vi "FeedbackDecode_20200902.vi"() -> ()   [LabVIEW 2016] (continued)
  T12 = cluster{"ExperimentDate":timestamp, "ImplantDate":timestamp, "CerebusFolder":string, "Experimenter":string, "PatientNumber":string, "DominantHand":string, "DeviceType":string, "DeviceSerial":string, "DeviceHemisphere":string, "DeviceRegion":string, "TaskType":string, "TaskComments":string, "RecordingComments":string, "GeneralObservations":string}
  T13 = typedef "FeedbackDecode_CogLoadClust.ctl" = cluster{"EEGTrigger":bool, "ConnectECG":bool, "TriggerECGwithTargets":bool, "SecondaryTask":bool, "MinTimeBetweenStimuli":dbl, "VariableTimeBetweenStimuli":dbl, "StimulusDuration":dbl}
  T14 = cluster{"[0]":u32, "[1]":u32, "[2]":u32, "[3]":u32}
  T15 = enum16{"---", "ReadMvnt", "WriteMvnt", "ReadEncode", "WriteEncode", "ReadDecode", "WriteDecode"}
  T16 = enum16{"Initialize", "Acquire Start", "Acquire Response", "Finalize"}
  T17 = enum8{"Enabled", "Disabled", "Disabled and Grayed Out"}
  T18 = enum16{"---", "Bakeoff11", "Bakeoff21", "Bakeoff31", "Bakeoff32", "LukeEmpty", "MPLEmpty", "MPLUnknown", "MPLBasic", "MPLTarg", "LukeBasic"}
  T19 = enum16{"Initialize", "Wait", "BuildInitStr", "BuildKalmanStr", "BuildStimStr", "BuildEMGStr", "GetEvent", "SendEvent", "ContIO", "LoadTrainFile", "CopyTraining", "Close"}
  T20 = cluster{"LV":cluster{"Name":string, "IP":string}, "ML":cluster{"Name":string, "IP":string}}
  T21 = enum32{"Invalid", "Standard", "Closed", "Hidden", "Minimized", "Maximized"}
  T22 = enum16{"open", "replace", "create", "open or create", "replace or create", "replace or create with confirmation"}
  T23 = enum16{"MSMS", "Bakeoff11", "Bakeoff21", "Bakeoff31", "Bakeoff32", "Bakeoff32_Ball", "Bakeoff32_Checkers", "Bakeoff32_Pen", "FragileBlock"}
  T24 = cluster{"MvntMat":dbl[][], "MvntName":string, "Tracking":enum8{"False", "True", "Mixed"}, "Radius":dbl}[]
  T25 = cluster{"Boolean 1":bool, "Boolean 2":bool, "Boolean 3":bool, "Boolean 4":bool, "Boolean 5":bool, "Boolean 6":bool, "Boolean 7":bool, "Boolean 8":bool, "Boolean 9":bool, "Boolean 10":bool, "Boolean 11":bool, "Boolean 12":bool, "Boolean 13":bool, "Boolean 14":bool, "Boolean 15":bool, "Boolean 16":bool, "Boolean 17":bool, "Boolean 18":bool, "Boolean 19":bool, "Boolean 20":bool, "Boolean 21":bool, "Boolean 22":bool, "Boolean 23":bool, "Boolean 24":bool, "Boolean 25":bool, "Boolean 26":bool, "Boolean 27":bool, "Boolean 28":bool, "Boolean 29":bool, "Boolean 30":bool, "Boolean 31":bool, "Boolean 32":bool, "Boolean 33":bool, "Boolean 34":bool, "Boolean 35":bool, "Boolean 36":bool, "Boolean 37":bool, "Boolean 38":bool, "Boolean 39":bool, "Boolean 40":bool, "Boolean 41":bool, "Boolean 42":bool, "Boolean 43":bool, "Boolean 44":bool, "Boolean 45":bool, "Boolean 46":bool, "Boolean 47":bool, "Boolean 48":bool, "Boolean 49":bool, "Boolean 50":bool, "Boolean 51":bool, "Boolean 52":bool, "Boolean 53":bool, "Boolean 54":bool, "Boolean 55":bool, "Boolean 56":bool, "Boolean 57":bool, "Boolean 58":bool, "Boolean 59":bool, "Boolean 60":bool, "Boolean 61":bool, "Boolean 62":bool, "Boolean 63":bool, "Boolean 64":bool, "Boolean 65":bool, "Boolean 66":bool, "Boolean 67":bool, "Boolean 68":bool, "Boolean 69":bool, "Boolean 70":bool, "Boolean 71":bool, "Boolean 72":bool, "Boolean 73":bool, "Boolean 74":bool, "Boolean 75":bool, "Boolean 76":bool, "Boolean 77":bool, "Boolean 78":bool, "Boolean 79":bool, "Boolean 80":bool, "Boolean 81":bool, "Boolean 82":bool, "Boolean 83":bool, "Boolean 84":bool, "Boolean 85":bool, "Boolean 86":bool, "Boolean 87":bool, "Boolean 88":bool, "Boolean 89":bool, "Boolean 90":bool, "Boolean 91":bool, "Boolean 92":bool, "Boolean 93":bool, "Boolean 94":bool, "Boolean 95":bool, "Boolean 96":bool, "Boolean 97":bool, "Boolean 98":bool, "Boolean 99":bool, "Boolean 100":bool}[]
  T26 = cluster{"[0]":dbl, "[1]":dbl, "[2]":dbl, "[3]":dbl, "[4]":dbl, "[5]":dbl, "[6]":dbl, "[7]":dbl, "[8]":dbl, "[9]":dbl, "[10]":dbl, "[11]":dbl}
  T27 = typedef "XDNodeRunTimeDep.lvlib/timing_clust.ctl" = cluster{"Expected End [f-1]":u64, "Actual End [f-1]":u64, "Finished Late? [f-1]":bool, "Expected End [i-1]":u64, "Actual End [i-1]":u64, "Finished Late? [i-1]":bool, "Expected Start [i]":u64, "Actual Start [i]":u64, "Expected Start [f]":u64, "Actual Start [f]":u64, "Source Name":string, "Structure Name":string, "Period":i64, "Deadline":i64, "Offset":i64, "Start":i64, "Priority":i32, "Timeout":i32, "Mode":T28, "Wakeup Reason":T29, "Error":errorcluster, "Source Type":string, "Secondary Source Type":string, "Global End Time":u64, "Global Start Time":u64, "Frame Duration":u64, "Iteration Duration":u64, "Assigned CPU":i32, "I/O Scan Engine Mode":u32}
  T28 = typedef "XDNodeRunTimeDep.lvlib/nitl_modes.ctl" = enum32{"No Change", "Process missed periods, maintain original phase", "Discard missed periods, maintain original phase", "Process missed periods, ignore original phase", "Discard missed periods, ignore original phase"}
  T29 = typedef "XDNodeRunTimeDep.lvlib/wakeup.ctl" = enum32{"Normal", "Aborted", "Asynchronous wakeup", "Timing source error", "Timed loop error", "Timeout"}
  T30 = enum16{"MSMS", "BakeOff1", "BakeOff2", "BakeOff3"}
  T31 = typedef "LVPositionTypeDef.ctl" = cluster{"Left":i32, "Top":i32}
  T32 = typedef "LVBoundsTypeDef.ctl" = cluster{"Width":u32, "Height":u32}
  T33 = cluster{cluster{"[0]":u32, "[1]":u32, "[2]":u32, "[3]":u32}, "HMSize":cluster{"NumCol":dbl, "NumRows":dbl}}
  T34 = cluster{"Left":i32, "Top":i32, "Width":u32, "Height":u32}
  T35 = cluster{"Name":string, "Type":string, "ID":string, "Num":string, "COM":dbl[], "Offset":dbl[], "RotationAxis":dbl[], "OrientationMatrix":dbl[][], "MinAngle":dbl, "MaxAngle":dbl, "InboardID":string, "InboardNum":string, "InboardCOM":dbl[], "OutboardID":string, "OutboardNum":string, "OutboardCOM":dbl[]}[]
  T36 = cluster{"ModelName":string, "Value":dbl[][], "CompNames":string[]}
  T37 = enum16{"Off", "Training", "Decode", "COB", "LEAP"}
  T38 = cluster{"ContMvntVal[0]":dbl, "ContMvntVal[1]":dbl, "ContMvntVal[2]":dbl, "ContMvntVal[3]":dbl, "ContMvntVal[4]":dbl, "ContMvntVal[5]":dbl, "ContMvntVal[6]":dbl, "ContMvntVal[7]":dbl, "ContMvntVal[8]":dbl, "ContMvntVal[9]":dbl, "ContMvntVal[10]":dbl, "ContMvntVal[11]":dbl}
  T39 = cluster{"ContTargetVal[0]":dbl, "ContTargetVal[1]":dbl, "ContTargetVal[2]":dbl, "ContTargetVal[3]":dbl, "ContTargetVal[4]":dbl, "ContTargetVal[5]":dbl, "ContTargetVal[6]":dbl, "ContTargetVal[7]":dbl, "ContTargetVal[8]":dbl, "ContTargetVal[9]":dbl, "ContTargetVal[10]":dbl, "ContTargetVal[11]":dbl}
  T40 = cluster{"LoopTimings":cluster{"MLCalcTime":dbl, "MLTotalTime":dbl}, "Kalman":cluster{"Thumb":dbl, "Index":dbl, "Middle":dbl, "Ring":dbl, "Little":dbl, "ThumbInt":dbl, "IndexInt":dbl, "RingInt":dbl, "LittleInt":dbl, "Wrist":dbl, "WristYaw":dbl, "WristRoll":dbl}, "Kinematics":cluster{"Thumb":dbl, "Index":dbl, "Middle":dbl, "Ring":dbl, "Little":dbl, "ThumbInt":dbl, "IndexInt":dbl, "RingInt":dbl, "LittleInt":dbl, "Wrist":dbl, "WristYaw":dbl, "WristRoll":dbl}, "ElectRates":dbl[], "SelWfs":dbl[][], "TrainCnt":dbl, "EMGPwr":dbl[], "SelData":cluster{dbl, dbl, "RasterOut":dbl[]}[], "SelRate":cluster{"CurIdx":dbl, dbl, "RasterOut":dbl[]}[], "SelKin":cluster{dbl, dbl, "RasterOut":dbl[]}[], "NIPTime":dbl, "VREID":i16, "StimWf":dbl[], "RawDecodeOutput":dbl[], "TASKA IR sensors":dbl[], "TASKA baro sensors":dbl[]}
  T41 = cluster{"Thumb":dbl, "Index":dbl, "Middle":dbl, "Ring":dbl, "Little":dbl, "ThumbInt":dbl, "IndexInt":dbl, "RingInt":dbl, "LittleInt":dbl, "Wrist":dbl, "WristYaw":dbl, "WristRoll":dbl}
  T42 = cluster{"Delay":dbl, "Rise":dbl, "Hold":dbl, "Trial":dbl}
  T43 = enum16{"Position", "Latching", "Leaky", "Velocity"}[]
  T44 = enum16{"Standard", "Mean", "Refit", "LinSVReg", "NonLinSVReg", "PCA", "DWPRR", "AdaptKF", "NN", "NN_python", "AdaptKF2", "KF_Short_Goal"}
  T45 = typedef "LVPoint32TypeDef.ctl" = cluster{"Horizontal":i32, "Vertical":i32}
  T46 = cluster{"KGain":sgl[][], "KMvnts":cluster{"Thumb":bool, "Index":bool, "Middle":bool, "Ring":bool, "Little":bool, "ThumbInt":bool, "IndexInt":bool, "RingInt":bool, "LittleInt":bool, "WristPitch":bool, "WristYaw":bool, "WristRoll":bool}, "KThresh":sgl[][], "CtrlMode":enum16{"Position", "Latching", "Leaky", "Velocity"}[], "CtrlSpd":sgl[]}
  T47 = enum16{"RMS Single", "RMS All", "RMS Auto", "Volt Single", "Volt All"}
  T48 = cluster{"[0]":bool, "[1]":bool, "[2]":bool, "[3]":bool, "[4]":bool, "[5]":bool, "[6]":bool, "[7]":bool, "[8]":bool, "[9]":bool, "[10]":bool, "[11]":bool, "[12]":bool, "[13]":bool, "[14]":bool, "[15]":bool, "[16]":bool, "[17]":bool, "[18]":bool, "[19]":bool, "[20]":bool, "[21]":bool, "[22]":bool, "[23]":bool, "[24]":bool, "[25]":bool, "[26]":bool, "[27]":bool, "[28]":bool, "[29]":bool, "[30]":bool, "[31]":bool, "[32]":bool, "[33]":bool, "[34]":bool, "[35]":bool, "[36]":bool, "[37]":bool, "[38]":bool, "[39]":bool, "[40]":bool, "[41]":bool, "[42]":bool, "[43]":bool, "[44]":bool, "[45]":bool, "[46]":bool, "[47]":bool, "[48]":bool, "[49]":bool, "[50]":bool, "[51]":bool, "[52]":bool, "[53]":bool, "[54]":bool, "[55]":bool, "[56]":bool, "[57]":bool, "[58]":bool, "[59]":bool, "[60]":bool, "[61]":bool, "[62]":bool, "[63]":bool, "[64]":bool, "[65]":bool, "[66]":bool, "[67]":bool, "[68]":bool, "[69]":bool, "[70]":bool, "[71]":bool, "[72]":bool, "[73]":bool, "[74]":bool, "[75]":bool, "[76]":bool, "[77]":bool, "[78]":bool, "[79]":bool, "[80]":bool, "[81]":bool, "[82]":bool, "[83]":bool, "[84]":bool, "[85]":bool, "[86]":bool, "[87]":bool, "[88]":bool, "[89]":bool, "[90]":bool, "[91]":bool, "[92]":bool, "[93]":bool, "[94]":bool, "[95]":bool, "[96]":bool, "[97]":bool, "[98]":bool, "[99]":bool}
  T49 = cluster{"[0]":bool, "[1]":bool, "[2]":bool, "[3]":bool, "[4]":bool, "[5]":bool, "[6]":bool, "[7]":bool, "[8]":bool, "[9]":bool, "[10]":bool, "[11]":bool, "[12]":bool, "[13]":bool, "[14]":bool, "[15]":bool, "[16]":bool, "[17]":bool, "[18]":bool, "[19]":bool, "[20]":bool, "[21]":bool, "[22]":bool, "[23]":bool, "[24]":bool, "[25]":bool, "[26]":bool, "[27]":bool, "[28]":bool, "[29]":bool, "[30]":bool, "[31]":bool, "[32]":bool, "[33]":bool, "[34]":bool, "[35]":bool, "[36]":bool, "[37]":bool, "[38]":bool, "[39]":bool, "[40]":bool, "[41]":bool, "[42]":bool, "[43]":bool, "[44]":bool, "[45]":bool, "[46]":bool, "[47]":bool, "[48]":bool, "[49]":bool, "[50]":bool, "[51]":bool, "[52]":bool, "[53]":bool, "[54]":bool, "[55]":bool, "[56]":bool, "[57]":bool, "[58]":bool, "[59]":bool, "[60]":bool, "[61]":bool, "[62]":bool, "[63]":bool, "[64]":bool, "[65]":bool, "[66]":bool, "[67]":bool, "[68]":bool, "[69]":bool, "[70]":bool, "[71]":bool, "[72]":bool, "[73]":bool, "[74]":bool, "[75]":bool, "[76]":bool, "[77]":bool, "[78]":bool, "[79]":bool}
  T50 = enum16{"Position", "Latching", "Leaky", "Velocity"}
  T51 = cluster{"Shift":bool, "Ctrl":bool, "Alt":bool, "Cmd":bool, "Opt":bool}
  T52 = cluster{"Region":bool, "Receptor":bool, "Electrode":bool, "Min Amp":bool, "Max Amp":bool, "Min Freq":bool, "Max Freq":bool, "Duration":bool}
  T53 = typedef "eventvkey.ctl" = enum16{"ASCII", "Enter", "Return", "Shift", "Ctrl", "Alt", "Cmd", "Opt", "Caps", "NumLock", "Clear", "Break", "Up", "Down", "Left", "Right", "Insert", "Delete", "Home", "End", "PageUp", "PageDown", "Escape", "Help", "Pause", "ScrollLock", "F1", "F2", "F3", "F4", "F5", "F6", "F7", "F8", "F9", "F10", "F11", "F12", "F13", "F14", "F15", "F16", "F17", "F18", "F19", "F20", "F21", "F22", "F23", "F24", "Play", "VolumeUp", "VolumeDown", "Mute", "Two Byte Char"}
  T54 = cluster{"Boolean 1":bool, "Boolean 2":bool, "Boolean 3":bool, "Boolean 4":bool, "Boolean 5":bool, "Boolean 6":bool, "Boolean 7":bool, "Boolean 8":bool, "Boolean 9":bool, "Boolean 10":bool, "Boolean 11":bool, "Boolean 12":bool, "Boolean 13":bool, "Boolean 14":bool, "Boolean 15":bool, "Boolean 16":bool, "Boolean 17":bool, "Boolean 18":bool, "Boolean 19":bool, "Boolean 20":bool, "Boolean 21":bool, "Boolean 22":bool, "Boolean 23":bool, "Boolean 24":bool, "Boolean 25":bool, "Boolean 26":bool, "Boolean 27":bool, "Boolean 28":bool, "Boolean 29":bool, "Boolean 30":bool, "Boolean 31":bool, "Boolean 32":bool, "Boolean 33":bool, "Boolean 34":bool, "Boolean 35":bool, "Boolean 36":bool, "Boolean 37":bool, "Boolean 38":bool, "Boolean 39":bool, "Boolean 40":bool, "Boolean 41":bool, "Boolean 42":bool, "Boolean 43":bool, "Boolean 44":bool, "Boolean 45":bool, "Boolean 46":bool, "Boolean 47":bool, "Boolean 48":bool, "Boolean 49":bool, "Boolean 50":bool, "Boolean 51":bool, "Boolean 52":bool, "Boolean 53":bool, "Boolean 54":bool, "Boolean 55":bool, "Boolean 56":bool, "Boolean 57":bool, "Boolean 58":bool, "Boolean 59":bool, "Boolean 60":bool, "Boolean 61":bool, "Boolean 62":bool, "Boolean 63":bool, "Boolean 64":bool, "Boolean 65":bool, "Boolean 66":bool, "Boolean 67":bool, "Boolean 68":bool, "Boolean 69":bool, "Boolean 70":bool, "Boolean 71":bool, "Boolean 72":bool, "Boolean 73":bool, "Boolean 74":bool, "Boolean 75":bool, "Boolean 76":bool, "Boolean 77":bool, "Boolean 78":bool, "Boolean 79":bool, "Boolean 80":bool, "Boolean 81":bool, "Boolean 82":bool, "Boolean 83":bool, "Boolean 84":bool, "Boolean 85":bool, "Boolean 86":bool, "Boolean 87":bool, "Boolean 88":bool, "Boolean 89":bool, "Boolean 90":bool, "Boolean 91":bool, "Boolean 92":bool, "Boolean 93":bool, "Boolean 94":bool, "Boolean 95":bool, "Boolean 96":bool, "Boolean 97":bool, "Boolean 98":bool, "Boolean 99":bool, "Boolean 100":bool}
  T55 = cluster{"[0]":bool, "[1]":bool, "[2]":bool, "[3]":bool, "[4]":bool, "[5]":bool, "[6]":bool, "[7]":bool, "[8]":bool, "[9]":bool, "[10]":bool, "[11]":bool, "[12]":bool, "[13]":bool, "[14]":bool, "[15]":bool, "[16]":bool, "[17]":bool, "[18]":bool, "[19]":bool, "[20]":bool, "[21]":bool, "[22]":bool, "[23]":bool, "[24]":bool, "[25]":bool, "[26]":bool, "[27]":bool, "[28]":bool, "[29]":bool, "[30]":bool, "[31]":bool, "[32]":bool, "[33]":bool, "[34]":bool, "[35]":bool, "[36]":bool, "[37]":bool, "[38]":bool, "[39]":bool, "[40]":bool, "[41]":bool, "[42]":bool, "[43]":bool, "[44]":bool, "[45]":bool, "[46]":bool, "[47]":bool, "[48]":bool, "[49]":bool, "[50]":bool, "[51]":bool, "[52]":bool, "[53]":bool, "[54]":bool, "[55]":bool, "[56]":bool, "[57]":bool, "[58]":bool, "[59]":bool, "[60]":bool, "[61]":bool, "[62]":bool, "[63]":bool, "[64]":bool, "[65]":bool, "[66]":bool, "[67]":bool, "[68]":bool, "[69]":bool, "[70]":bool, "[71]":bool, "[72]":bool, "[73]":bool, "[74]":bool, "[75]":bool, "[76]":bool, "[77]":bool, "[78]":bool, "[79]":bool, "[80]":bool, "[81]":bool, "[82]":bool, "[83]":bool, "[84]":bool, "[85]":bool, "[86]":bool, "[87]":bool, "[88]":bool, "[89]":bool, "[90]":bool, "[91]":bool, "[92]":bool, "[93]":bool, "[94]":bool, "[95]":bool, "[96]":bool, "[97]":bool, "[98]":bool, "[99]":bool}[]
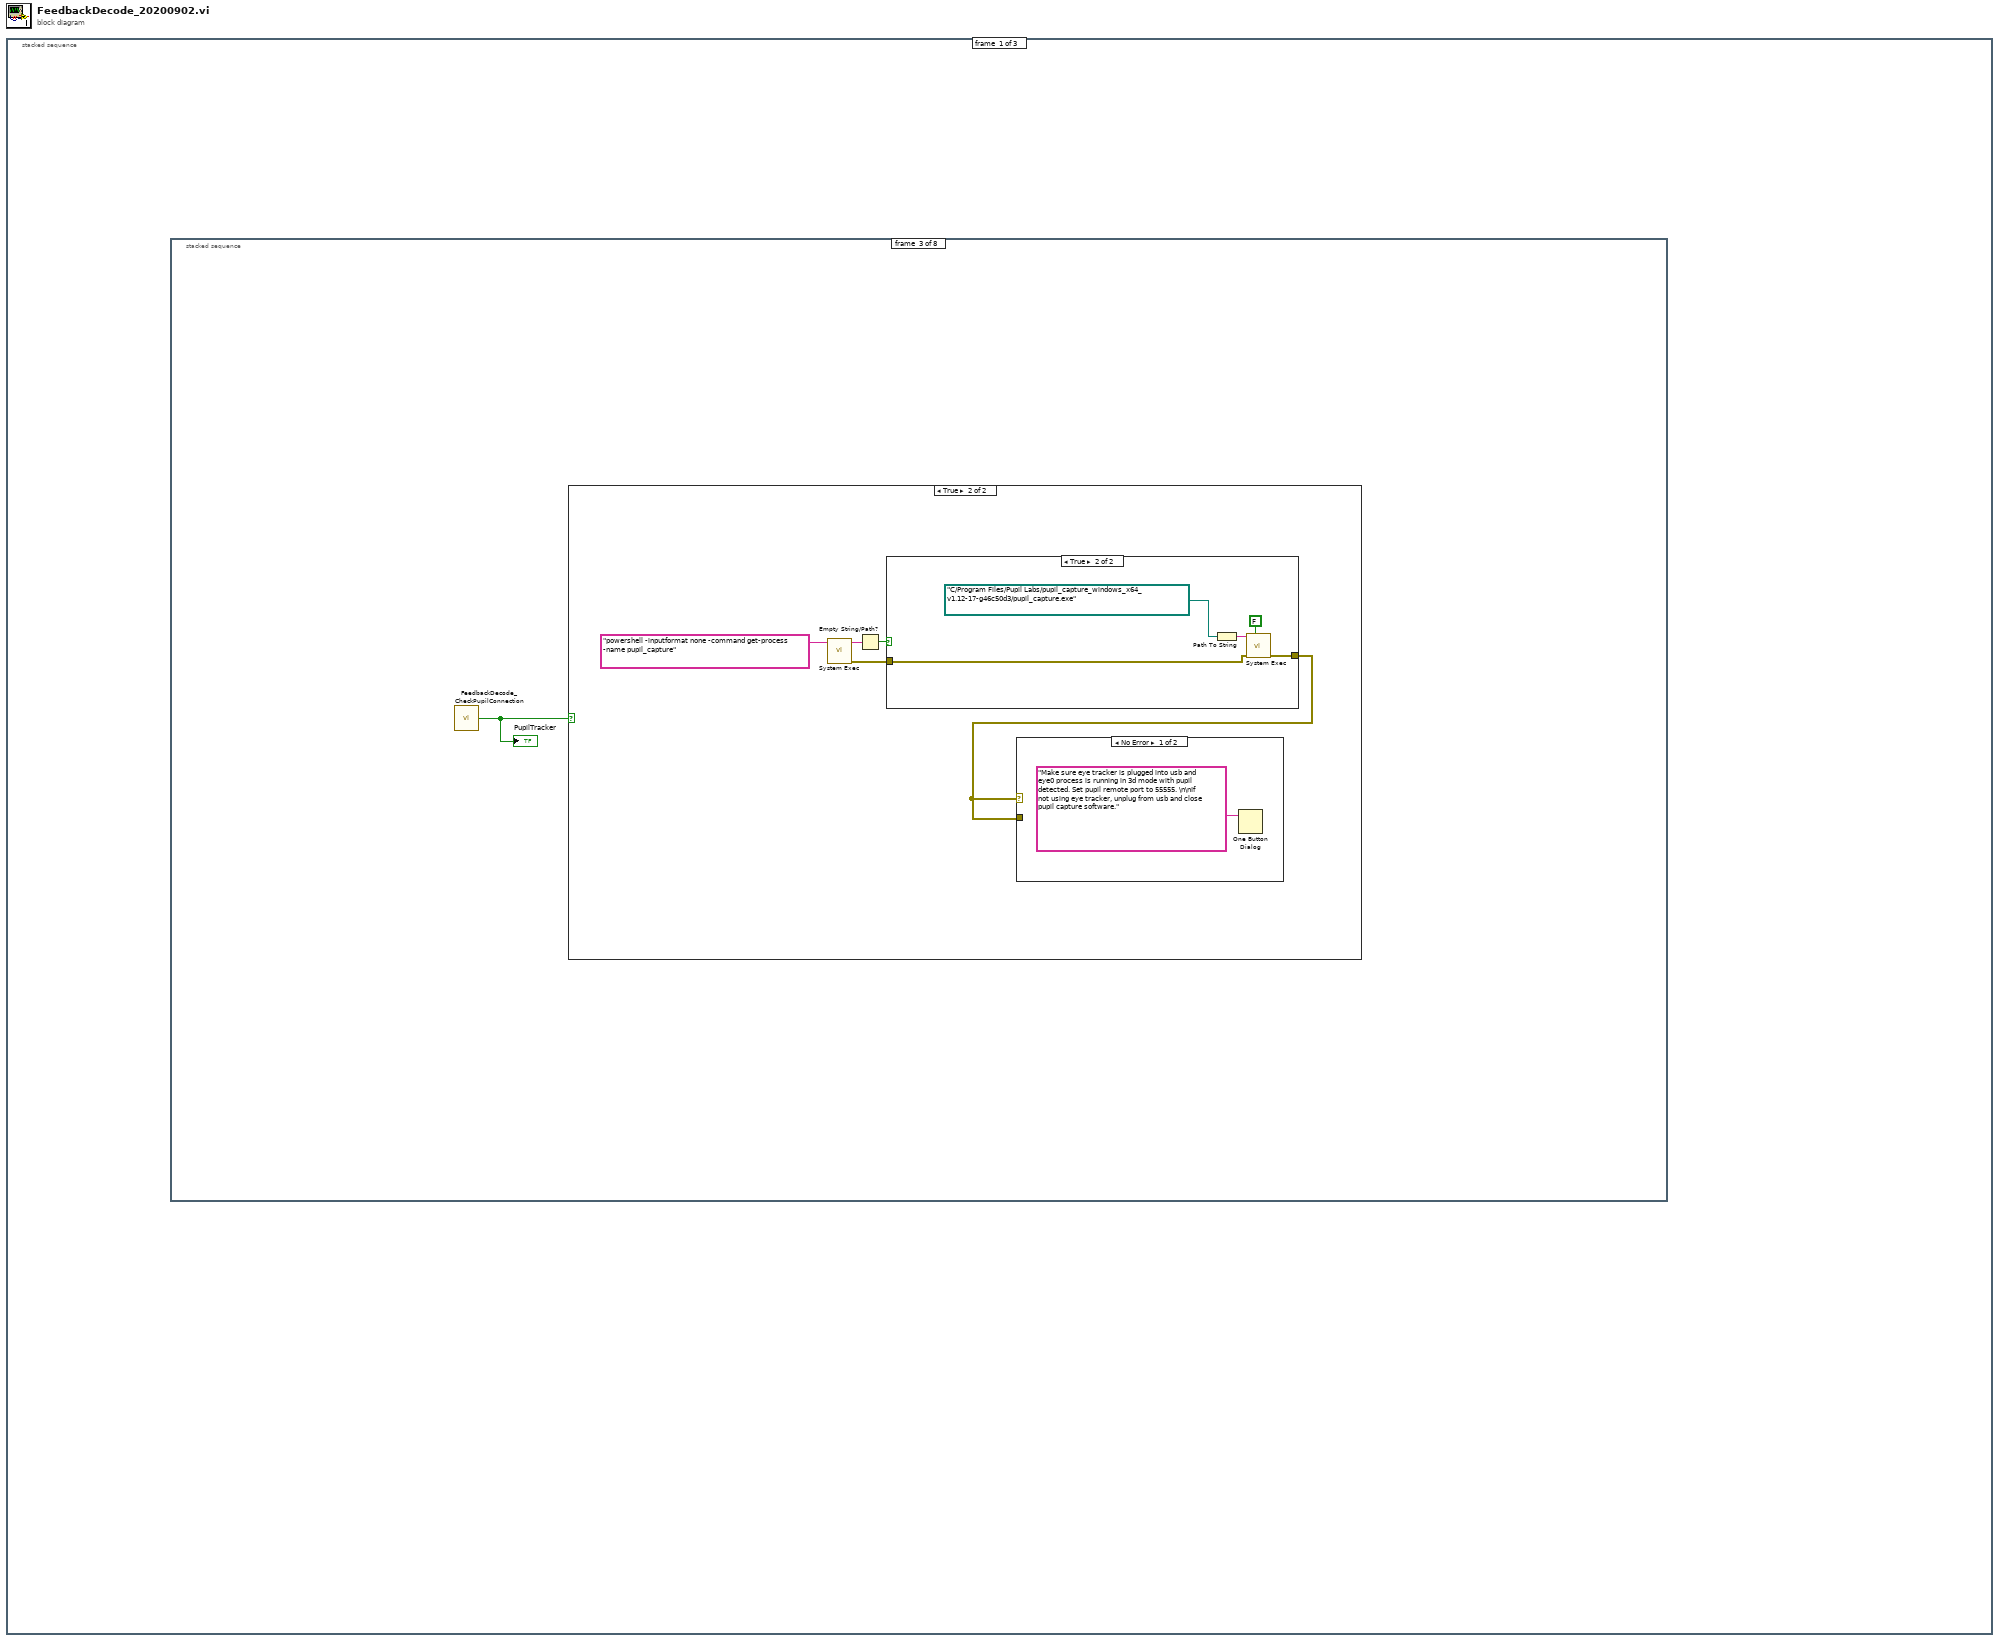
[diagram p0: block diagram]
diagram:
  n1 = stacked-sequence {
    frame #0 {
      n2 = stacked-sequence {
        frame #0 {
          w43 = FALSE ("Finished")
          w50 = 0.0  # MvntEvnt
          w66 = u64 0 ("BaseCnt1")
          w153 = enum16{"Initialize", "Reset", "Run"}."Initialize" ("Mode")
          w139 = "" ("TrialTypeStr")
          w120 = path "C:/Users/Administrator/Code/General/Databases/PatientDatabase.udl" ("DatabaseUDL")
          # "Is shared enabled?"
          # "TASKA"
          # "for analog sensors"
          n3 = local write "TASKASharedControlBeta"(0.0 ("TASKASharedControlBeta")) -> ()
          n4 = local write "Beta Mode"("Fixed" ("Beta Mode")) -> ()
          n5 = local write "Computer Goal"("Close" ("Computer Goal")) -> ()
          n6 = local write "TASKA Shared Control"(FALSE ("TASKA Shared Control")) -> ()
          n7 = property on="MedianHM" class="Pict"() -> ("Position"=w117:T31, "Draw Area Size"=w116:T32)  [unwired: 2 in, 2 out]
          n8 = property on="UlnarHM" class="Pict"() -> ("Position"=w112:T31, "Draw Area Size"=w113:T32)  [unwired: 2 in, 2 out]
          n9 = property on="EMGHM" class="Pict"() -> ("Position"=w98:T31, "Draw Area Size"=w97:T32)  [unwired: 2 in, 2 out]
          n10 = Initialize Array(0.0 ("element"), 496 ("dimension size")) -> (w52:dbl[])
          n11 = Cluster To Array(cluster=w117) -> (array=w146:i32[])
          n12 = Cluster To Array(cluster=w116) -> (array=w147:u32[])
          n13 = Cluster To Array(cluster=w112) -> (array=w111:i32[])
          n14 = Cluster To Array(cluster=w113) -> (array=w110:u32[])
          n15 = Cluster To Array(cluster=w98) -> (array=w99:i32[])
          n16 = Cluster To Array(cluster=w97) -> (array=w100:u32[])
          n17 = call "FeedbackDecode_AllEMGHM.vi"("Intensities"=w52, "Mode"=enum16{"Initialize", "Run"}."Initialize") -> ()  [unwired: 2 in]
          n18 = property on="Finished" class="Bool (strict)"("DisabledEnum"=T17."Disabled and Grayed Out" ("Disabled"), "Value"=w43, "Blinking"=w43) -> ()  [unwired: 2 in, 2 out]
          n19 = Build Array (concatenate)(w146, w147) -> (w148:u32[])
          n20 = Build Array (concatenate)(w111, w110) -> (w109:u32[])
          n21 = Build Array (concatenate)(w99, w100) -> (w101:u32[])
          n22 = mathscript code="GridArray = reshape(rot90(reshape(1:100,10,10),-1),1,100);"() -> ("GridArray"=→"UEAHMIdx":i32[])  [unwired: 1 in, 1 out]
          n23 = property on="ParamsTable" class="Arr (strict)"() -> ("Index Values"=w79:u32[], "Left"=w71:i32, "Width"=w70:u32)  [unwired: 2 in, 2 out]
          n24 = Array To Cluster(array=w148) -> (cluster=w149:T14)
          "MedianPos" <- w149
          n25 = Array To Cluster(array=w109) -> (cluster=w105:T14)
          "UlnarPos" <- w105
          n26 = Array To Cluster(array=w101) -> (cluster=w96:T14)
          "EMGPos" <- w96
          n27 = for {
            N: 2 -> [_]
            tunnel: [w178] -> w41 mode=indexing
            i -> [w177]
            n28 = case shown="0, Default" w177 {
              tunnel: [w179 w183] -> w178
              frame 0, Default {
                n29 = vi-ref "FeedbackDecode_PickROI.vi"() -> (w182:refnum<vi>)
                n30 = invoke class="VI" method="FP.Open"(reference=w182, "Activate"=TRUE ("Activate?"), "State"=T21."Hidden") -> (reference out=w179:refnum<vi>)  [unwired: 2 in, 4 out]
              }
              frame 1 {
                n31 = vi-ref "FeedbackDecode_PickROI_Adv.vi"() -> (w186:refnum<vi>)
                n32 = invoke class="VI" method="FP.Open"(reference=w186, "Activate"=TRUE ("Activate?"), "State"=T21."Hidden") -> (reference out=w183:refnum<vi>)  [unwired: 2 in, 4 out]
              }
            }
          }
          "RespRefArray" <- w41
          n33 = stacked-sequence {
            frame #0 {
              w169 = FALSE ("TASKA Reset Success")
              n34 = local write "TASKA Reset Success"(w169) -> ()
              n35 = local write "TASKA Reset Break"(w169) -> ()
              n36 = local write "TASKA Timer"(w169) -> ()
            }
            frame #1 {
              n37 = property on="TASKA Timer" class="Bool (strict)"("DisabledEnum"=T17."Enabled" ("Disabled")) -> ()  [unwired: 2 in, 2 out]
            }
          }
          n38 = Bundle(w149, "HMSize"="HMSize") -> (w150:T33)  [unwired: 1 in]
          n39 = Bundle(w105, "HMSize"="HMSize") -> (w106:T33)  [unwired: 1 in]
          n40 = Bundle(w96, "HMSize"="HMSize") -> (w104:T33)  [unwired: 1 in]
          n41 = call "FeedbackDecode_PlotHeatmap.vi"("InitCluster"=w150, "Instance"=0, "Mode"=enum16{"Initialize", "Run", "Mouse"}."Initialize") -> ("Pic"=→"MedianHM":picture, "CurrPos"=w90:i32)  [unwired: 3 in]
          "SelElect" <- w90
          n42 = call "FeedbackDecode_PlotHeatmap.vi"("InitCluster"=w106, "Instance"=1, "Mode"=enum16{"Initialize", "Run", "Mouse"}."Initialize") -> ("Pic"=→"UlnarHM":picture)  [unwired: 3 in, 1 out]
          n43 = call "FeedbackDecode_PlotHeatmap.vi"("InitCluster"=w104, "Instance"=2, "Mode"=enum16{"Initialize", "Run", "Mouse"}."Initialize") -> ("Pic"=→"EMGHM":picture)  [unwired: 3 in, 1 out]
          n44 = property on="Sel" class="Arr (strict)"("Index Values"=w79) -> ()  [unwired: 2 in, 2 out]
          n45 = Bundle("Left"=w71, "Width"=w70) -> (→"ParamsTableLoc":cluster{"Left":i32, "Width":u32})  [unwired: 1 in]
          n46 = disable-structure shown="Disabled" {
            frame Disabled {
              n47 = vi-ref "FeedbackDecode_MSMS2DEKA.vi"() -> (w176:refnum<vi>)
              n48 = invoke class="VI" method="FP.Open"(reference=w176, "Activate"=FALSE ("Activate?"), "State"=T21."Minimized") -> ()  [unwired: 2 in, 5 out]
            }
            frame Enabled {
            }
          }
          n49 = property on="KUEA" class="Clust (strict)"() -> ("Left"=w164:i32, "Top"=w163:i32, "Width"=w162:u32, "Height"=w161:u32)  [unwired: 2 in, 2 out]
          n50 = for {
            N: 80 -> [_]
            tunnel: [w190] -> w94 mode=indexing
            i -> [w191]
            n51 = Increment(x=w191) -> (x+1=w190:i32)
          }
          "EMGHMIdx" <- w94
          n52 = Initialize Array(0.0 ("element"), 100 ("dimension size")) -> (→"StimArray":dbl[])
          n53 = property class="VI"() -> ("Name"=→"TaskType":string)  [unwired: 2 in, 2 out]
          n54 = Bundle("Left"=w164, "Top"=w163, "Width"=w162, "Height"=w161) -> (w160:T34)  [unwired: 1 in]
          "HoverPicPos" <- w160
          n55 = call <vilib>:"Application Directory.vi"() -> ("Application Directory"=w29:path)
          n56 = call <vilib>:"Check if File or Folder Exists.vi"("path"=path "D:/") -> ("file or folder exists?"=w18:bool)  [unwired: 8 in, 2 out]
          n57 = vi-ref "FeedbackDecode_PlaySound.vi"() -> (w155:refnum<vi>)
          n58 = disable-structure shown="Disabled" {
            frame Disabled {
              n59 = vi-ref "FeedbackDecode_AllEMGHM.vi"() -> (w187:refnum<vi>)
              n60 = invoke class="VI" method="FP.Open"(reference=w187, "Activate"=FALSE ("Activate?"), "State"=T21."Minimized") -> ()  [unwired: 2 in, 5 out]
            }
            frame Enabled {
            }
          }
          n61 = Build Path(base path=w29, name or relative path="build") -> (appended path=w10:path)
          "BuildDir" <- w10
          n62 = call "FeedbackDecode_HoverElect.vi"("Border"=2.0, "PicPos"=w160, "Mode"=enum16{"Initialize", "Run"}."Initialize") -> ("Elect"=w141:i32)  [unwired: 3 in, 1 out]
          n63 = property class="VI"(reference=w155) -> ("Name"=w154:string)  [unwired: 1 in, 2 out]
          n64 = Select(t=path "D:/FeedbackDecode", s=w18, f=path "C:/Data/FeedbackDecode" ("path")) -> (s? t:f=w14:path)
          "DataDir" <- w14
          n65 = Unbundle By Name("DecodeClust") -> ("NumComp"=w23:enum16{"1 Computer", "2 Computers"})
          n66 = Path To String(path=w10) -> (string=w12:string)
          n67 = Path To String(path=w14) -> (string=w16:string)
          n68 = Unbundle By Name("MvntBuilder") -> ("Mode"=w34:enum16{"Selected", "Block", "Random"}, "NTrials"=w37:dbl, "MvntList"=w38:T24)
          n69 = property on="MvntList" class="Arr (strict)"() -> ("Index Values"=w40:u32[])  [unwired: 2 in, 2 out]
          n70 = Open VI Reference(type specifier VI Refnum (for type only)=refnum<vi> refnum ("application reference (local)"), vi path=w154, options=128) -> (vi reference=→"PSRef":refnum<vi>)  [unwired: 3 in, 1 out]
          n71 = Unbundle By Name("MvntBuilder") -> ("TargParams.Radius"=w85:dbl)
          n72 = Search and Replace String(input string=w12, search string=":", replace string="@" ("replace string (\"\")")) -> (result string=w9:string)  [unwired: 5 in, 3 out]
          n73 = Search and Replace String(input string=w16, search string=":", replace string="@" ("replace string (\"\")")) -> (result string=w8:string)  [unwired: 5 in, 3 out]
          n74 = case shown="\"1 Computer\"" w23 {
            tunnel: [T20 {"LV"={"Name"="PNILABVIEW", "IP"="155.100.90.215"}, "ML"={"Name"="PNIMATLAB", "IP"="155.100.90.185"}} ("CompID") T20 {"LV"={"Name"="PNILABVIEW", "IP"="127.0.0.1"}, "ML"={"Name"="PNIMATLAB", "IP"="127.0.0.2"}} ("CompID")] -> w22
            frame "2 Computers", Default {
            }
            frame "1 Computer" {
            }
          }
          n75 = Array Size(array=w38) -> (size(s)=w39:i32)
          n76 = Index Array(array=w40) -> (element=w36:u32)  [unwired: 1 in]
          n77 = call "FeedbackDecode_GenRandBlockIdxs2.vi"("Mode"=w34, "Reset"=TRUE, "NumTrials"=w37, "NumIdxs"=w39, "CurrIdx"=w36) -> ("Perc"=w32:dbl)  [unwired: 1 out]
          n78 = Initialize Array(0.0 ("element"), 2 ("dimension size"), 12 ("dimension size")) -> (w75:dbl[][])
          n79 = Bundle By Name(cluster="MvntBuilder", "PercTrials"=w32) -> (w31:T6)
          n80 = call "FeedbackDecode_RunOnce.vi"("Instance"=0, "Mode"=enum16{"Reset", "Run"}."Reset") -> ()  [unwired: 1 out]
          n81 = Bundle By Name(cluster="DecodeClust", "BuildDir"=w9, "DataDir"=w8, "TrainParams.TargRad"=w85, "DataFolder"="00000000-000000", "SelElect"=w90, "CompID"=w22, "HoverElect"=w141, "KinSrc"=enum16{"Off", "Training", "Decode", "COB"}."Off", "TrialCnt"=w75, "KDFFile"="") -> (w82:T5)
          n82 = Unbundle By Name(w22) -> ("LV.IP"=→"LVIP":string, "ML.IP"=→"MLIP":string)
          n83 = local write "MvntBuilder"(w31) -> ()
          n84 = call "FeedbackDecode_RunOnce.vi"("Instance"=1, "Mode"=enum16{"Reset", "Run"}."Reset") -> ()  [unwired: 1 out]
          n85 = call "FeedbackDecode_RunOnce.vi"("Instance"=2, "Mode"=enum16{"Reset", "Run"}."Reset") -> ()  [unwired: 1 out]
          n86 = global write "FeedbackDecode_Globals.vi" "FD_Stop"(FALSE ("EnablePtCtrl")) -> ()
          n87 = call "FeedbackDecode_MLComCtrl.vi"("CognitiveLoadIn"="CognitiveLoad", "DecodeClustIn"=w82, "EncodeClustIn"="EncodeClust", "Mode"=T19."Initialize") -> ("DecodeClustOut"=w30:T5, "EncodeClustOut"=w80:T9, "CognitiveLoadOut"=w1:T13)  [unwired: 4 in, 1 out]
          n88 = property class="DAQmx System"() -> ("DevNames"=w27:tag[])  [unwired: 2 in, 2 out]
          n89 = Unbundle By Name(w30) -> ("RasterWin"=w86:dbl)
          n90 = Unbundle By Name(w30) -> ("*Prosthesis"=w56:enum16{"MaleRight", "MaleLeft"})
          n91 = Create User Event(user event datatype=w50) -> (user event=w49:refnum<user-event>)  [unwired: 1 in, 1 out]
          "MvntEvnt" <- w49
          n92 = local write "EncodeClust"(w80) -> ()
          n93 = local write "CognitiveLoad"(w1) -> ()
          n94 = local write "DecodeClust"(w30) -> ()
          n95 = register-events(w49) -> (reference out=→"EvntReg":refnum<event-registration>)  [unwired: 2 in, 1 out]
          n96 = Divide(x=w86, y=0.033) -> (x/y=w83:dbl)
          n97 = Empty Array?(array=w27) -> (empty?=w26:bool)
          n98 = Format Into String(w56) -> (resulting string=w133:string)  [unwired: 3 in, 1 out]
          n99 = Multiply(x=2.0, y=w83) -> (x*y=w84:dbl)
          n100 = Not(x=w26) -> (.not. x?=→"DAQmx?":bool)
          n101 = property on="SelData" class="WFGraph (strict)"("XScale.Maximum"=w84) -> ()  [unwired: 2 in, 2 out]
          n102 = property on="SelRate" class="WFGraph (strict)"("XScale.Maximum"=w83) -> ()  [unwired: 2 in, 2 out]
          n103 = property on="SelKin" class="WFGraph (strict)"("XScale.Maximum"=w83) -> ()  [unwired: 2 in, 2 out]
          n104 = case shown="False" w26 {
            frame False {
              n105 = call <vilib>:"DAQmx Start Task.vi"("task/channels in"=refnum<k21> "AO0") -> ()  [unwired: 13 in, 2 out]
            }
            frame True {
            }
          }
          n106 = Concatenate Strings("C:\\Users\\Administrator\\Code\\General\\MSMS\\Scenarios\\", w133, "\\Model\\Prostheses\\prosthesis.xml") -> (w135:string)
          n107 = String To Path(string=w135) -> (path=w136:path)
          "XMLFile" <- w136
          n108 = call "FeedbackDecode_ParseMSMSXML.vi"("XMLFile"=w136) -> ("ComponentArray"=w130:T35)
          n109 = call "FeedbackDecode_UpdateDatabase.vi"("CallType"=enum16{"Initialize", "Save", "Load"}."Initialize", "DatabaseUDL"=w120) -> ("ExperimentDatesSorted"=w122:string[])  [unwired: 2 in, 2 out]
          n110 = call "FeedbackDecode_LoadMSMSParams.vi"("XMLFile"=w136) -> ("ModelParams"=w131:T36)  [unwired: 1 in]
          n111 = call "FeedbackDecode_SendMSMSPacket.vi"("CompArrayIn"=w130, "Mode"=enum16{"Initialize", "Run", "Close"}."Initialize") -> ()  [unwired: 5 in]
          n112 = property on="RecordSel" class="CmbBox"("Text.Text"="", "Strings[]"=w122) -> ()  [unwired: 2 in, 2 out]
          n113 = call "FeedbackDecode_BuildMSMSMvnt.vi"("CompArray"=w130, "ModelParams"=w131, "Mode"=enum16{"Initialize", "Run"}."Initialize") -> ()  [unwired: 4 in, 3 out]
          n114 = call "FeedbackDecode_GenContTarget.vi"("Mode"=w153) -> ()  [unwired: 5 in, 4 out]
          n115 = call "FeedbackDecode_GenContMvnt.vi"("Mode"=w153) -> ()  [unwired: 5 in, 3 out]
          n116 = call "FeedbackDecode_BuildMSMSSphere.vi"("CompArray"=w130, "ModelParams"=w131, "Mode"=enum16{"Initialize", "Run"}."Initialize") -> ()  [unwired: 4 in, 3 out]
          "State" <- T16."Initialize" ("Current State")
          "BaseCnt1" <- w66
          "TrialParameters" <- w139
          "DatabaseUDL" <- w120
          "TaskParameters" <- w139
          "Outcome" <- enum16{"---", "Success", "Failure"}."---" ("Outcome")
          "TrialArray" <- string[] [] ("TrialArray")
          "PrevIdx" <- 0.0 ("PrevIdx")
          "BaseCnt2" <- w66
          "TrainCnt" <- 0.0 ("TrainCnt")
          "Status" <- enum16{"In", "Out"}."Out" ("Status")
          "FileIO" <- T15."---" ("FileIO")
          "TargDist" <- dbl[] [0.0, 0.0, 0.0, 0.0, 0.0, 0.0] ("TargDist")
          "iTiming" <- "Timing"
          "NIPTime" <- 0.0 ("TrainCnt")
          "VRELabel" <- T18."---" ("VRELabel")
          "BaseCnt3" <- -inf
          "PulseStim" <- FALSE ("PulseStim")
          "RespStr" <- ""
          "StimCmd" <- ""
          "SelTog" <- FALSE ("SelTog")
          "StimTog" <- FALSE ("StimTog")
          "CurrMvnt" <- T1 {"MvntMat"=[], "MvntName"="", "Tracking"=enum."False", "Radius"=0.15} ("CurrMvnt")
        }
        frame #1 {
          # "Open Trellis if it is not already running"
          n117 = call <vilib>:"System Exec.vi"("command line"="powershell -inputformat none -command get-process -name Trellis") -> ("error out"=w240:errorcluster, "standard output"=w242:string)  [unwired: 7 in, 2 out]
          n118 = Empty String/Path?(string/path=w242) -> (empty?=w241:bool)
          n119 = case shown="True" w241 {
            tunnel: [w244 w246] -> w239
            tunnel: w240 -> [w244 w245]
            frame False {
            }
            frame True {
              n120 = Path To String(path=path "C:/Program Files (x86)/Ripple/Trellis/Apps/Trellis/bin/start_Trellis.bat") -> (string=w249:string)
              n121 = call <vilib>:"System Exec.vi"("wait until completion? (T)"=FALSE, "error in (no error)"=w245, "working directory"=path "C:/Program Files (x86)/Ripple/Trellis/Apps/Trellis/bin", "command line"=w249) -> ("error out"=w246:errorcluster)  [unwired: 4 in, 3 out]
            }
          }
          n122 = case shown="No Error" w239 {
            tunnel: w239 -> [_ w252]
            frame No Error {
              n123 = One Button Dialog(message="Load Trellis config file, enable appropriate channels for saving to disk, set file save directory to \"D:\\\", and make sure digital triggering is enabled.\n\nDigital Triggering...\nStart: Parallel (0x007F; 0x0011)\nStop: Parallel (0x007F; 0x0012) ") -> ()  [unwired: 1 in, 1 out]
            }
            frame Error {
              n124 = call <vilib>:"Simple Error Handler.vi"("error in (no error)"=w252) -> ()  [unwired: 4 in, 5 out]
            }
          }
        }
        frame #2 {
          n125 = call "FeedbackDecode_CheckPupilConnection.vi"() -> ("Connected?"=w253:bool)  [unwired: 1 in]
          "PupilTracker" <- w253
          n126 = case shown="True" w253 {
            frame False {
            }
            frame True {
              n127 = call <vilib>:"System Exec.vi"("command line"="powershell -inputformat none -command get-process -name pupil_capture") -> ("error out"=w255:errorcluster, "standard output"=w257:string)  [unwired: 7 in, 2 out]
              n128 = Empty String/Path?(string/path=w257) -> (empty?=w256:bool)
              n129 = case shown="True" w256 {
                tunnel: [w259 w261] -> w254
                tunnel: w255 -> [w259 w260]
                frame False {
                }
                frame True {
                  n130 = Path To String(path=path "C:/Program Files/Pupil Labs/pupil_capture_windows_x64_v1.12-17-g46c50d3/pupil_capture.exe") -> (string=w263:string)
                  n131 = call <vilib>:"System Exec.vi"("wait until completion? (T)"=FALSE, "error in (no error)"=w260, "command line"=w263) -> ("error out"=w261:errorcluster)  [unwired: 5 in, 3 out]
                }
              }
              n132 = case shown="No Error" w254 {
                tunnel: w254 -> [_ w266]
                frame No Error {
                  n133 = One Button Dialog(message="Make sure eye tracker is plugged into usb and eye0 process is running in 3d mode with pupil detected. Set pupil remote port to 55555. \n\nIf not using eye tracker, unplug from usb and close pupil capture software.") -> ()  [unwired: 1 in, 1 out]
                }
                frame Error {
                  n134 = call <vilib>:"Simple Error Handler.vi"("error in (no error)"=w266) -> ()  [unwired: 4 in, 5 out]
                }
              }
            }
          }
        }
        frame #3 {
          # "Create data folder and start params txt files"
          n135 = Get Date/Time In Seconds() -> (seconds since 1Jan1904=w284:timestamp)
          "ExperimentDate" <- w284
          n136 = local read "DataDir"() -> (w272:path)
          n137 = Format Date/Time String(time format string (%c)="%Y%m%d-%H%M%S", seconds (now)=w284) -> (date/time string=w267:string)  [unwired: 1 in]
          n138 = Build Path(base path=w272, name or relative path=w267) -> (appended path=w271:path)
          n139 = call <vilib>:"Check if File or Folder Exists.vi"("path"=w271) -> ("error out"=w270:errorcluster, "file or folder exists?"=w268:bool, "dup path"=w269:path)  [unwired: 8 in]
          n140 = case shown="False" w268 {
            tunnel: [w288 w290] -> w274
            tunnel: [w287 w289] -> w275
            tunnel: w270 -> [w286 w289]
            tunnel: w269 -> [w285 w290]
            frame False {
              n141 = Create Folder(path (use dialog)=w285, error in=w286) -> (created path=w288:path, error out=w287:errorcluster)  [unwired: 1 in, 1 out]
            }
            frame True {
            }
          }
          "DataPath" <- w274
          n142 = local read "DecodeClust"() -> (w273:T5)
          n143 = Bundle By Name(cluster=w273, "DataFolder"=w267) -> (w282:T5)
          n144 = local write "DecodeClust"(w282) -> ()
          n145 = Concatenate Strings("EventParams_" ("name or relative path"), w267, ".txt" ("string")) -> (w276:string)
          n146 = Build Path(base path=w274, name or relative path=w276) -> (appended path=w280:path)
          n147 = Open/Create/Replace File(file path (use dialog)=w280, error in=w275, operation (0:open)=T22."replace or create") -> (refnum out=→"EventParamsFID":refnum<file>)  [unwired: 3 in, 2 out]
        }
        frame #4 {
          # "start matlab executable on remote computer"
          n148 = local read "DecodeClust"() -> (w293:T5)
          n149 = Unbundle By Name(w293) -> ("StartML"=w292:bool, "NumComp"=w291:enum16{"1 Computer", "2 Computers"})
          n150 = case shown="True" w292 {
            tunnel: w291 -> [_ w294]
            frame False {
            }
            frame True {
              n151 = case shown="\"1 Computer\"" w294 {
                frame "1 Computer" {
                  n152 = local read "BuildDir"() -> (w295:path)
                  n153 = call <vilib>:"System Exec.vi"("wait until completion? (T)"=FALSE, "working directory"=w295, "command line"="cmd /c FeedbackDecode.exe 127.0.0.1") -> ()  [unwired: 5 in, 4 out]
                }
                frame "2 Computers", Default {
                  n154 = local read "TaskType"() -> (w301:string)
                  n155 = Search and Replace String(input string=w301, search string=".vi", replace string=".exe" ("replace string (\"\")")) -> (result string=w302:string)  [unwired: 5 in, 3 out]
                  n156 = local read "MLIP"() -> (w300:string)
                  n157 = local read "LVIP"() -> (w299:string)
                  n158 = Build Path(base path=path "D:/RemoteRepo", name or relative path=w302) -> (appended path=w303:path)
                  n159 = call "FeedbackDecode_RunProgram_PSExec.vi"("ProgramInput"=w299, "Program"=w303, "ComputerName"=w300, "Mode"=enum16{"Start", "Stop"}."Start") -> ()  [unwired: 1 out]
                }
              }
            }
          }
        }
        frame #5 {
          # "Wait for matlab to startup"
          n160 = call "FeedbackDecode_MLComCtrl.vi"("Mode"=T19."Wait") -> ()  [unwired: 7 in, 4 out]
        }
        frame #6 {
          # "MP: Added CL here"
          # "Send initialization variables to matlab"
          n161 = local read "CognitiveLoad"() -> (w310:T13)
          n162 = local read "EncodeClust"() -> (w319:T9)
          n163 = local read "DecodeClust"() -> (w320:T5)
          n164 = call "FeedbackDecode_MLComCtrl.vi"("CognitiveLoadIn"=w310, "DecodeClustIn"=w320, "EncodeClustIn"=w319, "Mode"=T19."BuildInitStr") -> ("DecodeClustOut"=w316:T5, "EncodeClustOut"=w317:T9, "CognitiveLoadOut"=w309:T13)  [unwired: 4 in, 1 out]
          n165 = Unbundle By Name(w316) -> ("EventStr"=w314:string, "NumComp"=→"NumComp":enum16{"1 Computer", "2 Computers"})
          n166 = call "FeedbackDecode_MLComCtrl.vi"("CognitiveLoadIn"=w309, "DecodeClustIn"=w316, "EncodeClustIn"=w317, "Mode"=T19."SendEvent") -> ("DecodeClustOut"=w321:T5, "EncodeClustOut"=w318:T9, "CognitiveLoadOut"=w308:T13)  [unwired: 4 in, 1 out]
          n167 = Concatenate Strings("InitParameters:" ("string"), w314) -> (w312:string)
          n168 = local read "EventParamsFID"() -> (w315:refnum<file>)
          n169 = local write "CognitiveLoad"(w308) -> ()
          n170 = local write "EncodeClust"(w318) -> ()
          n171 = local write "DecodeClust"(w321) -> ()
          n172 = call "FeedbackDecode_WriteTextEOL.vi"("text"=w312, "refnum in"=w315) -> ()  [unwired: 8 in, 2 out]
        }
        frame #7 {
          # "wait for matlab"
          n173 = call "FeedbackDecode_MLComCtrl.vi"("Mode"=T19."Wait") -> ()  [unwired: 7 in, 4 out]
        }
      }
    }
    frame #1 {
      n174 = node-c288() -> (w328:T27)  [unwired: 4 in]
      n175 = disable-structure shown="Disabled" {
        frame Disabled {
          n176 = while {
            stop <- w333 stop-if-true
            n177 = Wait (ms)(milliseconds to wait=u32 100) -> ()  [unwired: 1 out]
            n178 = global read "FeedbackDecode_Globals.vi" "FD_Stop"() -> (w333:bool)
            n179 = call "FeedbackDecode_DEKAHandCtrl.vi"("RunMode"=enum16{"Manual", "Decode"}."Decode") -> ()  [unwired: 1 in]
          }
        }
        frame Enabled {
        }
      }
      n180 = timed-loop {
        timing: w328 -> [_]
        timing-out: [_] -> w327
        i -> [w3318]
        stop <- w3200 stop-if-true
        w3251 = enum16{"Initialize", "Run", "Mouse"}."Run" ("Mode")
        n181 = node-c288() -> (w3322:i64, w3319:i64)  [unwired: 1 in]
        "LoopPeriod" <- w3322
        n182 = local read "DecodeClust"() -> (w3209:T5)
        n183 = local read "ManualClust"() -> (w3204:T7)
        n184 = global read "FeedbackDecode_Globals.vi" "FD_Force"() -> (w3192:dbl[])
        n185 = local read "prevWAVChart"() -> (w3305:dbl[])
        n186 = global read "FeedbackDecode_Globals.vi" "FD_WAVChart"() -> (w3306:dbl[])
        n187 = local read "LoopCnt"() -> (w3303:u64)
        n188 = local read "LoopCnt"() -> (w3309:u64)
        n189 = local read "BaseCnt1"() -> (w3279:u64)
        n190 = local read "BaseCnt2"() -> (w3277:u64)
        n191 = local read "LoopCnt"() -> (w3190:u64)
        n192 = To Time Stamp(1:w3190) -> (0:w3179:timestamp)
        n193 = for {
          tunnel: w3192 -> [w3348] mode=indexing
          tunnel: [w3347] -> w3191 mode=indexing
          tunnel: w3179 -> [w3346]
          n194 = Build Array(w3348) -> (w3349:dbl[])
          n195 = Bundle By Name("Y"=w3349, "t0"=w3346) -> (w3347:waveform(dbl))  [unwired: 1 in]
        }
        "AnlgPlot" <- w3191
        n196 = local read "CurrMvnt"() -> (w3297:T1)
        n197 = Unbundle By Name(w3297) -> ("MvntMat"=w3296:dbl[][])
        n198 = Unbundle By Name(w3209) -> ("KinSrc"=w3207:T37)
        n199 = Not Equal?(x=w3305, y=w3306) -> (x != y?=w3307:bool[])
        n200 = call "FeedbackDecode_GenContMvnt.vi"("Mode"=enum16{"Initialize", "Reset", "Run"}."Run", "LoopCount"=w3303) -> ("ContMvntVal"=w3268:dbl[])  [unwired: 4 in, 2 out]
        n201 = call "FeedbackDecode_GenContTarget.vi"("LoopCount"=w3309, "Mode"=enum16{"Initialize", "Reset", "Run"}."Run") -> ("ContSphereVal"=w3312:dbl[][], "ContTargetVal"=w3222:dbl[])  [unwired: 4 in, 2 out]
        n202 = Add(x=w3279, y=u64 10) -> (x+y=w3281:u64)
        n203 = Add(x=w3277, y=u64 10) -> (x+y=w3275:u64)
        n204 = To Double Precision Float(number=w3322) -> (double precision float=w3321:dbl)
        n205 = To Double Precision Float(number=w3319) -> (double precision float=w3320:dbl)
        n206 = Or Array Elements(Boolean array=w3307) -> (logical OR=w3308:bool)
        n207 = Equal?(x=w3190, y=w3281) -> (x = y?=w3282:bool)
        n208 = Equal?(x=w3190, y=w3275) -> (x = y?=w3274:bool)
        n209 = global read "FeedbackDecode_Globals.vi" "FD_DEKAsensors"() -> (w3189:dbl[])
        n210 = Array To Cluster(array=w3268) -> (cluster=w3232:T38)
        n211 = Index Array(array=w3296, index (col)=0 ("disabled index (col)")) -> (element=w3294:dbl[])  [unwired: 1 in]
        n212 = case shown="True" w3308 {
          tunnel: w3306 -> [_ w3409]
          frame False {
          }
          frame True {
            "prevWAVChart" <- w3409
            "WAVChart" <- w3409
          }
        }
        n213 = case shown="True" w3282 {
          frame False {
          }
          frame True {
            n214 = local write "ResetCorr"(FALSE ("ResetCorr")) -> ()
          }
        }
        n215 = case shown="True" w3274 {
          frame False {
          }
          frame True {
            n216 = local read "DecodeClust"() -> (w3398:T5)
            n217 = Bundle By Name(cluster=w3398, "ClearWfs"=FALSE) -> (w3400:T5)
            n218 = local write "DecodeClust"(w3400) -> ()
          }
        }
        n219 = expression code="x/1000"(w3321) -> (w3324:dbl)
        n220 = expression code="x/1000"(w3320) -> (w3323:dbl)
        n221 = Absolute Value(x=w3294) -> (abs(x)=w3293:dbl[])
        n222 = Array Size(array=w3268) -> (size(s)=w3289:i32)
        n223 = case shown="\"Off\", Default" w3207 {
          tunnel: [w3406 w3407 w3408] -> w3300
          tunnel: w3232 -> [_ w3407 _]
          tunnel: w3204 -> [w3406 _ w3408]
          frame "Off", Default {
          }
          frame "Training" {
          }
          frame "COB" {
          }
        }
        n224 = Greater Than 0?(x=w3293) -> (x > 0?=w3292:bool[])
        n225 = Bundle(w3324, w3323) -> (→"LVTiming":cluster{dbl, dbl})  [unwired: 1 in]
        n226 = Search 1D Array(1D array=w3292, element=TRUE) -> (index of element=w3284:i32)  [unwired: 1 in]
        n227 = local read "TargDist"() -> (w3261:dbl[])
        n228 = local read "State"() -> (w3325:T16)
        n229 = local read "State"() -> (w3262:T16)
        n230 = Array To Cluster(array=w3222) -> (cluster=w3301:T39)
        n231 = local read "ManualDOF"() -> (w3203:T8)
        n232 = local read "EncodeClust"() -> (w3214:T9)
        n233 = local read "DekaSensorBreakThreshold"() -> (w3185:dbl[])
        n234 = for {
          tunnel: w3189 -> [w3338] mode=indexing
          tunnel: [w3342] -> w3188 mode=indexing
          tunnel: w3179 -> [w3341]
          tunnel: w3185 -> [w3340] mode=indexing
          tunnel: [w3339] -> w3184 mode=indexing
          # "convert sensor (0 to 1) to Newtons"
          n235 = Multiply(x=w3338, y=25.5) -> (x*y=w3336:dbl)
          n236 = Greater Or Equal?(x=w3336, y=w3340) -> (x >= y?=w3339:bool)
          n237 = Build Array(w3336) -> (w3343:dbl[])
          n238 = Bundle By Name("Y"=w3343, "t0"=w3341) -> (w3342:waveform(dbl))  [unwired: 1 in]
        }
        "DekaSensors" <- w3188
        n239 = Bundle By Name(cluster=w3209, "State"=w3262, "TargDist"=w3261, "Kinematics"=w3300, "Targets"=w3301) -> (w3263:T5)
        n240 = feedback #1() -> (w3283:dbl[])  [unwired: 1 in]
        n241 = local read "PltMode"() -> (w3259:enum16{"Rate", "Corr"})
        n242 = call "FeedbackDecode_MLComCtrl.vi"("DecodeClustIn"=w3263, "EncodeClustIn"=w3214, "Mode"=T19."GetEvent") -> ("DecodeClustOut"=w3217:T5, "EncodeClustOut"=w3216:T9)  [unwired: 5 in, 2 out]
        n243 = call "FeedbackDecode_MLComCtrl.vi"("DecodeClustIn"=w3217, "EncodeClustIn"=w3216, "ManualDOF"=w3203, "Mode"=T19."ContIO") -> ("DecodeClustOut"=w3215:T5, "EncodeClustOut"=w3213:T9, "MLClust"=w3302:T40)  [unwired: 4 in, 1 out]
        n244 = Unbundle By Name(w3215) -> ("EvntFlag"=w3233:bool, "TrainParams.Lag"=w3288:dbl)
        n245 = case shown="True" w3233 {
          tunnel: w3215 -> [_ w3391]
          tunnel: w3213 -> [_ w3390]
          frame False {
          }
          frame True {
            n246 = Bundle By Name(cluster=w3391, "EvntFlag"=FALSE) -> (w3392:T5)
            n247 = local write "DecodeClust"(w3392) -> ()
            n248 = call "FeedbackDecode_RunOnce.vi"("Instance"=2, "Mode"=enum16{"Reset", "Run"}."Reset") -> ()  [unwired: 1 out]
            n249 = local write "EncodeClust"(w3390) -> ()
          }
        }
        n250 = local read "EMGHMIdx"() -> (w3243:i32[])
        n251 = local read "UEAHMIdx"() -> (w3247:i32[])
        n252 = local read "StimArray"() -> (w3242:dbl[])
        n253 = Unbundle By Name(w3302) -> ("TASKA baro sensors"=w3178:dbl[], "TASKA IR sensors"=w3177:dbl[], "RawDecodeOutput"=w3187:dbl[], "StimWf"=→"StimWfGraph":dbl[], "Kalman"=w3231:T41, "TrainCnt"=w3267:dbl, "LoopTimings"=→"MLTiming":cluster{"MLCalcTime":dbl, "MLTotalTime":dbl}, "SelData"=→"SelData":cluster{dbl, dbl, "RasterOut":dbl[]}[], "SelWfs"=→"SelWfs":dbl[][], "ElectRates"=w3260:dbl[], "EMGPwr"=w3196:dbl[], "SelRate"=→"SelRate":cluster{"CurIdx":dbl, dbl, "RasterOut":dbl[]}[], "SelKin"=→"SelKin":cluster{dbl, dbl, "RasterOut":dbl[]}[], "NIPTime"=w3194:dbl, "VREID"=w3212:i16)
        n254 = call "FeedbackDecode_displayDecodeOutput.vi"("Input"=w3187) -> ()
        n255 = local write "VRELabel"(w3212) -> ()
        n256 = local write "TrainCnt"(w3267) -> ()
        n257 = local read "DAQmx?"() -> (w3181:bool)
        n258 = Index Array(array=w3222) -> (element=w3221:dbl)  [unwired: 1 in]
        n259 = disable-structure shown="Disabled" {
          disable-tunnel: w3196 -> [w3345 _]
          frame Disabled {
            n260 = call "FeedbackDecode_AllEMGHM.vi"("Intensities"=w3345, "Mode"=enum16{"Initialize", "Run"}."Run") -> ()  [unwired: 2 in]
          }
          frame Enabled {
          }
        }
        n261 = local write "NIPTime"(w3194) -> ()
        n262 = global write "FeedbackDecode_Globals.vi" "FD_NIPTime"(w3194) -> ()
        n263 = case shown="True" w3181 {
          tunnel: w3221 -> [_ w3333]
          frame False {
          }
          frame True {
            n264 = call-poly <vilib>:"DAQmx Write.vi"("task/channels in"=refnum<k21> "AO0", "data"=w3333) -> ()  [unwired: 11 in, 3 out]
          }
        }
        n265 = Array Subset(array=w3196, length=80) -> (w3197:dbl[])  [unwired: 1 in]
        n266 = Or Array Elements(Boolean array=w3184) -> (logical OR=w3183:bool)
        n267 = global read "FeedbackDecode_Globals.vi" "FD_AVIImage"() -> (→"AVIImage":T10)
        n268 = global read "FeedbackDecode_Globals.vi" "FD_FrameCount"() -> (→"FrameCount":i32)
        n269 = global read "FeedbackDecode_Globals.vi" "FD_SkippedFrames"() -> (→"SkippedFrames":i32)
        n270 = Build Array (concatenate)(w3260, w3197) -> (w3258:dbl[])
        n271 = call "FeedbackDecode_PtPtCorr.vi"("Rates"=w3258, "Initialize"="ResetCorr", "Training"=w3268, "Lag"=w3288) -> ("Corr"=w3287:dbl[])  [unwired: 1 in, 2 out]
        n272 = Reshape Array(w3287, 280.0 ("y"), w3289) -> (w3290:dbl[][])
        n273 = case shown="True" "HoldCorr" {
          tunnel: [w3404 w3405] -> w3257
          tunnel: w3290 -> [w3403 _]
          tunnel: w3284 -> [w3402 _]
          tunnel: w3283 -> [_ w3405]
          frame False {
            n274 = Index Array(array=w3403, index (col)=w3402) -> (element=w3404:dbl[])  [unwired: 1 in]
          }
          frame True {
          }
        }
        n275 = feedback-in #1(w3257) -> ()
        n276 = case shown="\"Rate\", Default" w3259 {
          tunnel: w3258 -> [w3395 _]
          tunnel: w3257 -> [_ w3397]
          tunnel: [w3395 w3397] -> w3244
          tunnel: ["HeatMap Range" cluster{"Min":dbl, "Max":dbl} {"Min"=0.0, "Max"=1.0} ("Range")] -> w3234
          frame "Rate", Default {
          }
          frame "Corr" {
          }
        }
        n277 = Array Subset(array=w3244, length=100) -> (w3241:dbl[])  [unwired: 1 in]
        n278 = Array Subset(array=w3244, index=100 ("length"), length=100) -> (w3240:dbl[])
        n279 = Array Subset(array=w3244, index=200 ("length"), length=80) -> (w3239:dbl[])
        n280 = Build Array(w3247, w3241, w3242) -> (w3246:dbl[][])
        n281 = Build Array(w3247, w3240, w3242) -> (w3245:dbl[][])
        n282 = Build Array(w3243, w3239, w3242) -> (w3238:dbl[][])
        n283 = call "FeedbackDecode_PlotHeatmap.vi"("Range"=w3234, "GridIntensity"=w3246, "Instance"=0, "Mode"=w3251) -> ("Pic"=w3237:picture)  [unwired: 2 in, 1 out]
